vi "Anritsu VNA Filter Unmeasurable Measurements.vi"(7 "Anritsu VNA":T5, 8 "error in (no error)":errorcluster, 10 "Parameters to Measure":T1[](array[typedef]) {"Channel" min=1 max=99 step=1; "Parameter"."Stimulus Port" min=1 step=1; "Parameter"."Response Port" min=1 step=1}, 11 "VISA Resource Name":refnum<visa-resource-name>) -> (0 "error out":errorcluster, 1 "Removed Parameters":T1[](array[typedef]) {"Channel" min=1 max=99 step=1; "Parameter"."Stimulus Port" min=1 step=1; "Parameter"."Response Port" min=1 step=1}, 2 "Filtered Parameters to Measure":T1[](array[typedef]) {"Channel" min=1 max=99 step=1; "Parameter"."Stimulus Port" min=1 step=1; "Parameter"."Response Port" min=1 step=1}, 3 "dup VISA Resource Name":refnum<visa-resource-name>, 4 "Measurements Removed?":bool)   [LabVIEW 2011]
uses:
  tests/S Parameter/TypeDefs/SP Parameter to Measure.ctl
  tests/S Parameter/TypeDefs/SP Parameter.ctl
  tests/S Parameter/TypeDefs/SP Calibration State.ctl
  tests/S Parameter/TypeDefs/SP Measurement Format.ctl
  TypeDefs/Anritsu VNA Instrument Info.ctl
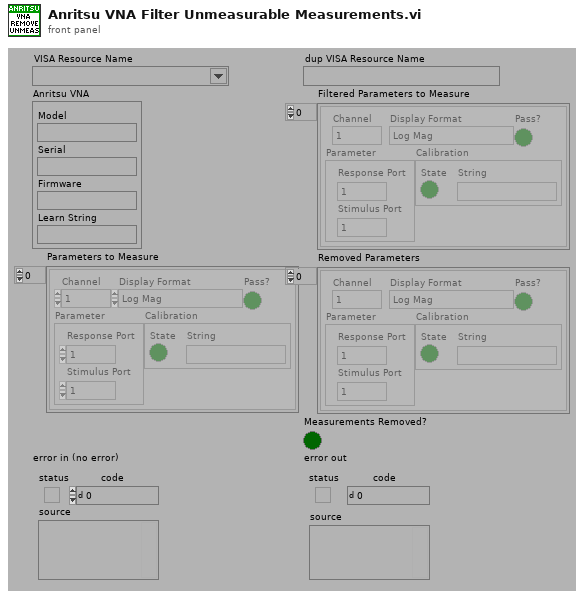
[diagram p1: front panel]
types:
  T1 = typedef "SP Parameter to Measure.ctl" = cluster{"Channel":i8, "Parameter":T2, "Calibration":T3, "Display Format":T4, "Pass?":bool}
  T2 = typedef "SP Parameter.ctl" = cluster{"Stimulus Port":i8, "Response Port":i8}
  T3 = typedef "SP Calibration State.ctl" = cluster{"State":bool, "String":string}
  T4 = typedef "SP Measurement Format.ctl" = enum32{"Log Mag", "Phase", "Delay", "Smith (R+jX)", "Polar (Re/Im)", "Linear Mag", "SWR", "Real", "Imaginary", "Smith (Lin/Phase)", "Smith (Log/Phase)", "Smith (Real/Imag)", "Smith (G+jB)", "Polar (Lin/Phase)", "Polar (Log/Phase)", "Expanded Phase", "Positive Phase", "Inverted Smith", "Unwrapped Phase", "Power Out", "Power In", "Linear Mag/Phase", "Log Mag/Phase", "Real/Imaginary"}
  T5 = typedef "Anritsu VNA Instrument Info.ctl" = cluster{"Model":string, "Serial":string, "Firmware":string, "Learn String":string}
  T6 = typedef "Anritsu VNA Model.ctl" = enum16{"Not Supported", "37XXXX", "MS20XXX", "MS462XX", "MS464XX"}
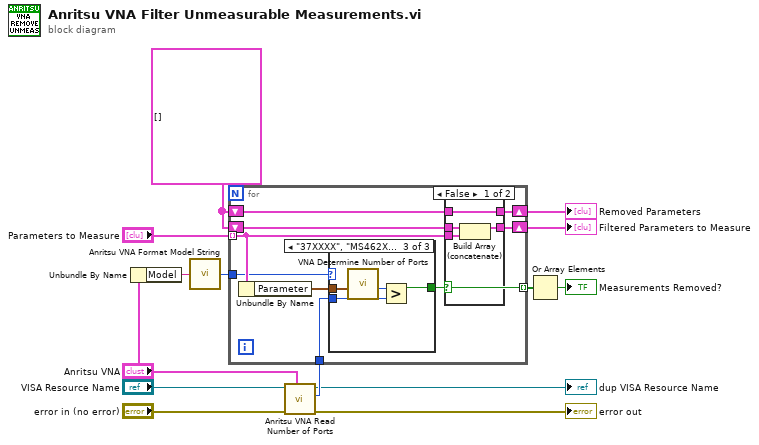
[diagram p0: block diagram]
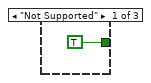
[diagram p2: hidden frame]
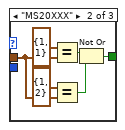
[diagram p3: hidden frame]
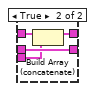
[diagram p4: hidden frame]
diagram:
  w6 = T1[] [] ("Parameters to Measure")
  n1 = Unbundle By Name("Anritsu VNA") -> ("Model"=w2:string)
  n2 = call "Anritsu VNA Format Model String.vi"("Model"=w2) -> ("Model"=w1:T6)
  n3 = call "Anritsu VNA Read Number of Ports.vi"("Anritsu VNA"="Anritsu VNA", "error in (no error)"="error in (no error)", "VISA Resource Name"="VISA Resource Name") -> ("error out"=→"error out":errorcluster, "Number of Ports"=w11:i8, "dup VISA Resource Name"=→"dup VISA Resource Name":refnum<visa-resource-name>)  [unwired: 6 out]
  n4 = for {
    tunnel: "Parameters to Measure" -> [w22] mode=indexing
    shift-right: [w21] -> w8
    shift-left: w6 -> [w23]
    tunnel: w11 -> [w19]
    tunnel: w1 -> [w18]
    shift-right: [w16] -> w5
    shift-left: w6 -> [w17]
    tunnel: [w15] -> w4 mode=indexing
    n5 = Unbundle By Name(w22) -> ("Parameter"=w20:T2)
    n6 = case shown="\"37XXXX\", \"MS462XX\", \"MS464XX\"" w18 {
      tunnel: w20 -> [_ w26 w33]
      tunnel: w19 -> [_ _ w32]
      tunnel: [TRUE w25 w31] -> w15
      frame "Not Supported" {
      }
      frame "MS20XXX" {
        n7 = Equal?(x=T2 {"Stimulus Port"=1, "Response Port"=1} ("Parameter"), y=w26) -> (x = y?=w29:bool)
        n8 = Equal?(x=T2 {"Stimulus Port"=1, "Response Port"=2} ("Parameter"), y=w26) -> (x = y?=w30:bool)
        n9 = Not Or(1:w30, 2:w29) -> (0:w25:bool)
      }
      frame "37XXXX", "MS462XX", "MS464XX" {
        n10 = call "VNA Determine Number of Ports.vi"("Parameter"=w33) -> ("Number of Ports"=w34:i8)  [unwired: 10 out]
        n11 = Greater?(x=w34, y=w32) -> (0:w31:bool)
      }
    }
    n12 = case shown="False" w15 {
      tunnel: w23 -> [w38 w42]
      tunnel: w22 -> [w37 w39]
      tunnel: [w36 w42] -> w21
      tunnel: w17 -> [w35 w41]
      tunnel: [w35 w40] -> w16
      frame False {
        n13 = Build Array (concatenate)(w38, w37) -> (w36:T1[])
      }
      frame True {
        n14 = Build Array (concatenate)(w41, w39) -> (w40:T1[])
      }
    }
  }
  "Filtered Parameters to Measure" <- w8
  "Removed Parameters" <- w5
  n15 = Or Array Elements(Boolean array=w4) -> (logical OR=→"Measurements Removed?":bool)
